vi "1A Read Sensor Data.vi"(8 "error (in)":errorcluster, 11 "VISA resource name (in)":refnum<visa-resource-name>="COM1") -> (0 "error (out)":errorcluster, 3 "VISA resource name (out)":refnum<visa-resource-name>)   [LabVIEW 2013]
doc: "This VI reads one sentence of data from the serial port associated with the WeatherStation Sensor (which must have been initialized previously using the \"1A Helper - Init Sensor.vi\"). \n\nIt reads one byte at a time, first waiting for the \"$\" (indicating the start of a sentence), then saving all bytes until a \"*ss\" is reached (the checksum, indicating the end of a sentence)."
uses:
  2-Think/2 Globals/2 Global.vi
  2-Think/2 Typedefs/indicator LED.ctl
panel:
  out "NMEA sentence":string
  out "Current Status":enum16{"Waiting", "Reading", "Time Out!"}(ring)
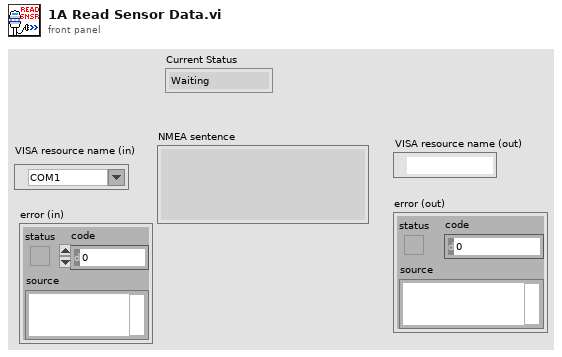
[diagram p1: front panel]
types:
  T1 = typedef "indicator LED.ctl" = bool
  T2 = typedef "generalized sensor status.ctl" = cluster{"Sensor Connected":T1, "Sensor Initialized":T1, "Sensor OK":T1, "Latest Error String":string, "GPS Lock":T1}
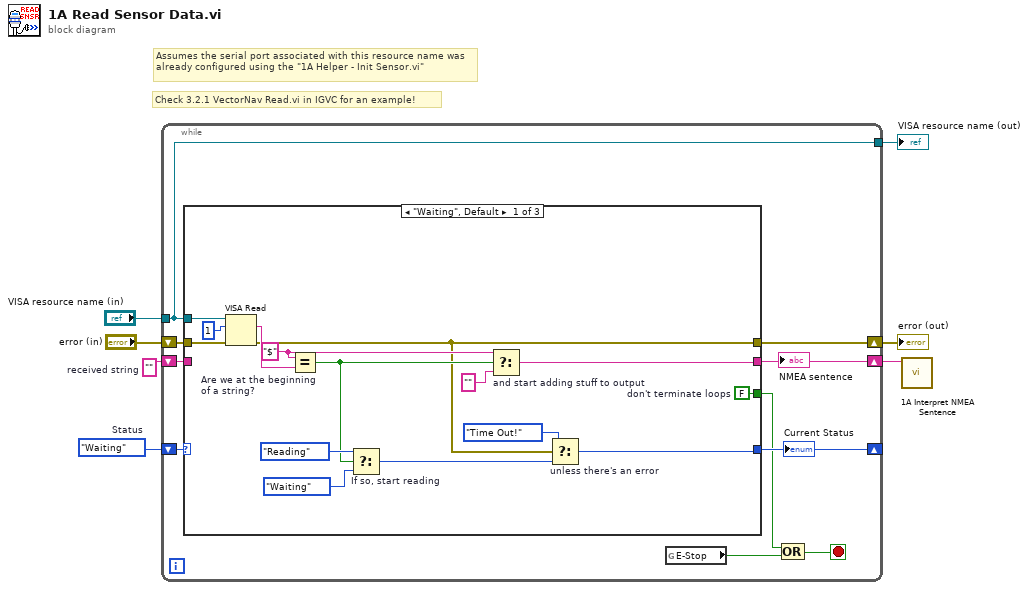
[diagram p0: block diagram]
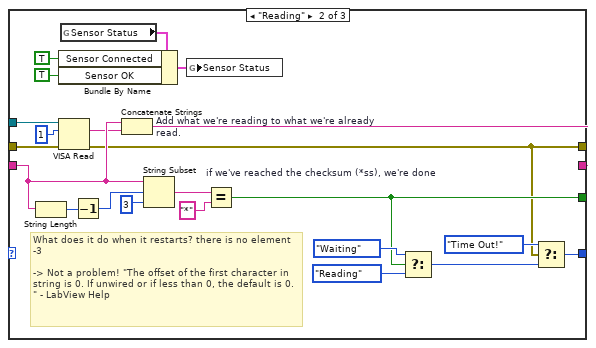
[diagram p2: hidden frame]
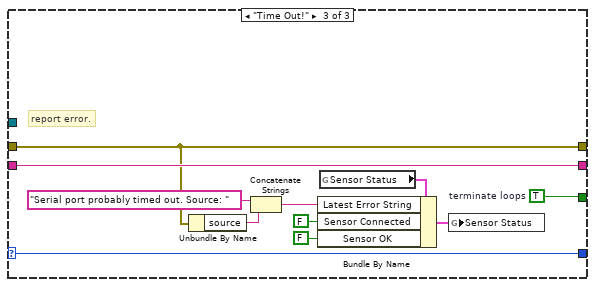
[diagram p3: hidden frame]
diagram:
  w4 = enum16{"Waiting", "Reading", "Time Out!"}."Waiting"  # Status
  w5 = ""  # received string
  # "Assumes the serial port associated with this resource name was already configured using the \"1A Helper - Init Sensor.vi\""
  # "Check 3.2.1 VectorNav Read.vi in IGVC for an example!"
  n1 = while {
    shift-right: [w10] -> w1
    shift-left: w5 -> [w17]
    shift-right: [w14] -> _
    shift-left: w4 -> [w16]
    tunnel: "VISA resource name (in)" -> [w9]
    shift-right: [w12] -> w2
    shift-left: "error (in)" -> [w13]
    tunnel: [w9] -> w3
    stop <- w15 stop-if-true
    n2 = case shown="\"Waiting\", Default" w16 {
      selector: w16 -> [_ _ w65]
      tunnel: w17 -> [_ w48 w64]
      tunnel: [w18 w54 w64] -> w10
      tunnel: [w23 w41 w65] -> w14
      tunnel: w9 -> [w26 w44 _]
      tunnel: w13 -> [w24 w42 w55]
      tunnel: [w21 w33 w55] -> w12
      tunnel: [w19 w38 w63] -> w11
      frame "Waiting", Default {
        w19 = FALSE  # don't terminate loops
        w28 = "$" ("x")
        n3 = VISA Read(VISA resource name=w26, byte count=u32 1, error in (no error)=w24) -> (read buffer=w27:string, error out=w21:errorcluster)  [unwired: 2 out]
        n4 = Equal? "Are we at the beginning of a string?"(x=w28, y=w27) -> (x = y?=w29:bool)
        n5 = Select "If so, start reading"(t=enum16{"Waiting", "Reading", "Time Out!"}."Reading", s=w29, f=enum16{"Waiting", "Reading", "Time Out!"}."Waiting" ("Current Status")) -> (s? t:f=w22:enum16{"Waiting", "Reading", "Time Out!"})
        n6 = Select "and start adding stuff to output"(t=w28, s=w29, f="") -> (s? t:f=w18:string)
        n7 = Select "unless there's an error"(t=enum16{"Waiting", "Reading", "Time Out!"}."Time Out!", s=w21, f=w22) -> (s? t:f=w23:enum16{"Waiting", "Reading", "Time Out!"})
      }
      frame "Reading" {
        # "What does it do when it restarts? there is no element -3\n\n-> Not a problem! \"The offset of the first character in string is 0. If unwired or if less than 0, the default is 0. \" - LabView Help"
        n8 = String Length(string=w48) -> (length=w53:i32)
        n9 = VISA Read(VISA resource name=w44, byte count=u32 1, error in (no error)=w42) -> (read buffer=w47:string, error out=w33:errorcluster)  [unwired: 2 out]
        n10 = global read "2 Global.vi" "Sensor Status"() -> (w34:T2)
        n11 = Bundle By Name(cluster=w34, "Sensor Connected"=T1 TRUE, "Sensor OK"=T1 TRUE) -> (w35:T2)
        n12 = Decrement(x=w53) -> (x-1=w52:i32)
        n13 = Concatenate Strings "Add what we're reading to what we're already read."(w48, w47) -> (w54:string)
        n14 = String Subset(string=w48, offset (0)=w52, length (rest)=3 ("length (rest)")) -> (substring=w50:string)
        n15 = global write "2 Global.vi" "Sensor Status"(w35) -> ()
        n16 = Equal? "if we've reached the checksum (*ss), we're done"(x=w50, y="*") -> (x = y?=w38:bool)
        n17 = Select(t=enum16{"Waiting", "Reading", "Time Out!"}."Waiting", s=w38, f=enum16{"Waiting", "Reading", "Time Out!"}."Reading" ("Status")) -> (s? t:f=w40:enum16{"Waiting", "Reading", "Time Out!"})
        n18 = Select(t=enum16{"Waiting", "Reading", "Time Out!"}."Time Out!", s=w33, f=w40) -> (s? t:f=w41:enum16{"Waiting", "Reading", "Time Out!"})
      }
      frame "Time Out!" {
        w63 = TRUE  # terminate loops
        # "report error."
        n19 = Unbundle By Name(w55) -> ("source"=w62:string)
        n20 = Concatenate Strings("Serial port probably timed out. Source: " ("string"), w62) -> (w61:string)
        n21 = global read "2 Global.vi" "Sensor Status"() -> (w56:T2)
        n22 = Bundle By Name(cluster=w56, "Latest Error String"=w61, "Sensor Connected"=T1 FALSE, "Sensor OK"=T1 FALSE) -> (w57:T2)
        n23 = global write "2 Global.vi" "Sensor Status"(w57) -> ()
      }
    }
    "Current Status" <- w14
    "NMEA sentence" <- w10
    n24 = global read "2 Global.vi" "E-Stop"() -> (w8:bool)
    n25 = Compound Arithmetic op=OR(w11, w8) -> (w15:bool)
  }
  "VISA resource name (out)" <- w3
  "error (out)" <- w2
  n26 = call "1A Interpret NMEA Sentence.vi"("NMEA Sentence"=w1) -> ()  [unwired: 11 in]
